vi "(2) Built In Homing Function - Just X.vi"() -> ()   [LabVIEW 2020]
uses:
  <instrlib>/Arcus Ethernet Driver 1.0.0/ArcusEthernetComm/classes/Controller/_Controller.lvclass
panel:
  in  "Home":bool
  out "Scanning Rig Disconnection":errorcluster={"status"=TRUE, "code"=0, "source"=""}
  in  "error in (no error)":errorcluster
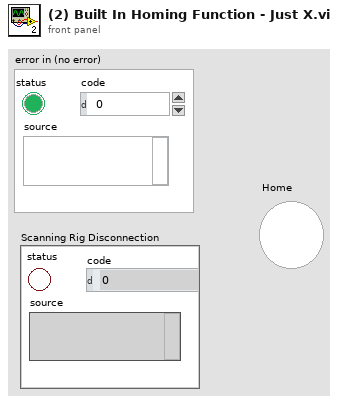
[diagram p1: front panel]
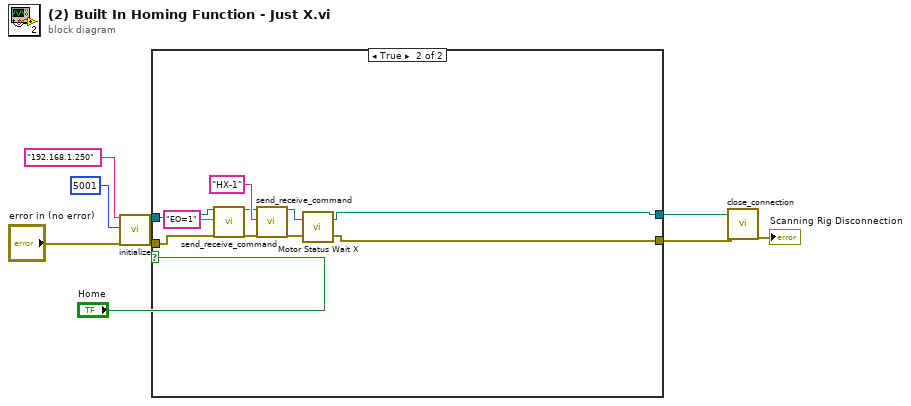
[diagram p0: block diagram]
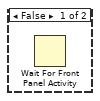
[diagram p2: hidden frame]
diagram:
  n1 = call <instrlib>:"initialize.vi"("ip_address (in)"="192.168.1.250", "dev_port(def=5001)"=u16 5001, "error in (no error)"="error in (no error)") -> ("reference (out)"=w5:refnum<class "_Controller.lvclass">, "error out"=w4:errorcluster)  [unwired: 15 in]
  n2 = case shown="True" "Home" {
    tunnel: w5 -> [_ w13]
    tunnel: w4 -> [_ w12]
    tunnel: [_ w10] -> w2
    tunnel: [_ w11] -> w1
    frame False {
      n3 = Wait For Front Panel Activity() -> ()  [unwired: 3 in, 1 out]
    }
    frame True {
      n4 = call <instrlib>:"send_receive_command.vi"("reference (in)"=w13, "ASCII Command (in)"="EO=1", "error in (no error)"=w12) -> ("reference (out)"=w15:refnum<class "_Controller.lvclass">, "error out"=w14:errorcluster)  [unwired: 12 in, 3 out]
      n5 = call <instrlib>:"send_receive_command.vi"("reference (in)"=w15, "ASCII Command (in)"="HX-1", "error in (no error)"=w14) -> ("reference (out)"=w18:refnum<class "_Controller.lvclass">, "error out"=w17:errorcluster)  [unwired: 12 in, 3 out]
      n6 = call "Motor Status Wait X.vi"("error in"=w17, "reference (in)"=w18) -> ("error out"=w10:errorcluster, "reference (out)"=w11:refnum<class "_Controller.lvclass">)
    }
  }
  n7 = call <instrlib>:"close_connection.vi"("reference (in)"=w1, "error in (no error)"=w2) -> ("error out"=→"Scanning Rig Disconnection":errorcluster)  [unwired: 16 in, 1 out]
